vi "ex_FindNextAvailFile.vi"(8 "error in":errorcluster, 11 "desired file path":path) -> (0 "error out":errorcluster, 3 "next avail file path":path)   [LabVIEW 2020]
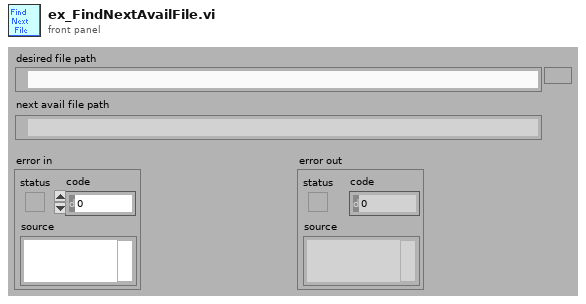
[diagram p1: front panel]
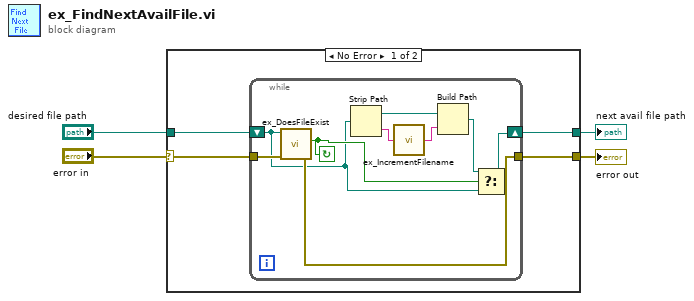
[diagram p0: block diagram]
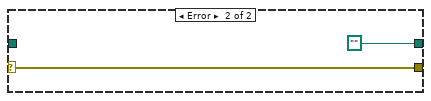
[diagram p2: hidden frame]
diagram:
  n1 = case shown="No Error" "error in" {
    selector: "error in" -> [w8 w19]
    tunnel: [w7 w19] -> w3
    tunnel: "desired file path" -> [w5 _]
    tunnel: [w6 path ""] -> w1
    frame No Error {
      n2 = while {
        tunnel: w8 -> [w17]
        shift-right: [w14] -> w6
        shift-left: w5 -> [w13]
        tunnel: [w16] -> w7
        stop <- w15 continue-if-true
        n3 = call "ex_DoesFileExist.vi"("error in"=w17, "file path"=w13) -> ("error out"=w16:errorcluster, "file exists"=w15:bool)  [unwired: 4 out]
        n4 = Strip Path(path=w13) -> (stripped path=w10:path, name=w12:string)
        n5 = call "ex_IncrementFilename.vi"("name base"=w12) -> ("new name"=w11:string)  [unwired: 4 out]
        n6 = Build Path(base path=w10, name or relative path=w11) -> (appended path=w9:path)
        n7 = Select(t=w9, s=w15, f=w13) -> (s? t:f=w14:path)
      }
    }
    frame Error {
    }
  }
  "error out" <- w3
  "next avail file path" <- w1
